vi "startReadSetDuration.vi"(8 "error in (no error)":errorcluster, 9 "duration":dbl, 10 "ElectrometerController in":refnum<class "ElectrometerController.lvclass">, 11 "State in":refnum<class "State.lvclass">) -> (0 "error out":errorcluster, 2 "ElectrometerController. out":refnum<class "ElectrometerController.lvclass">, 3 "State out":refnum<class "State.lvclass">)   [LabVIEW 2016, in "State.lvclass"]
uses:
  State.lvclass
  ElectrometerController/ElectrometerController.lvclass
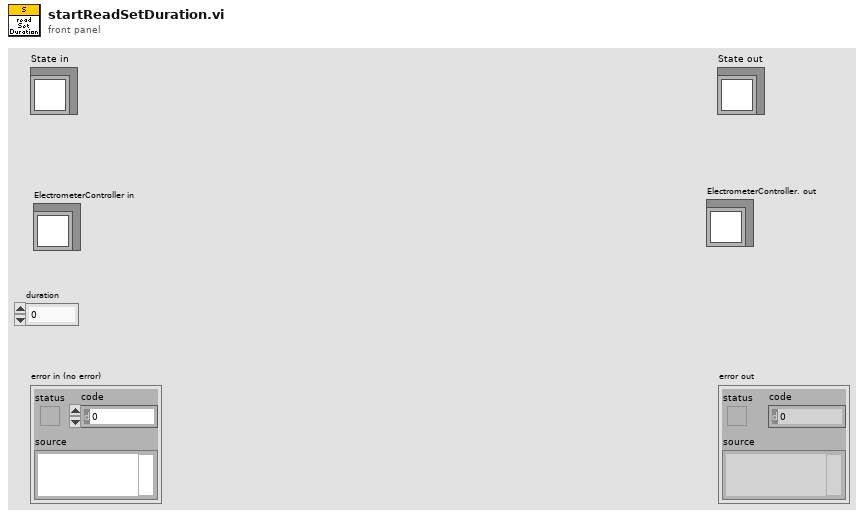
[diagram p1: front panel]
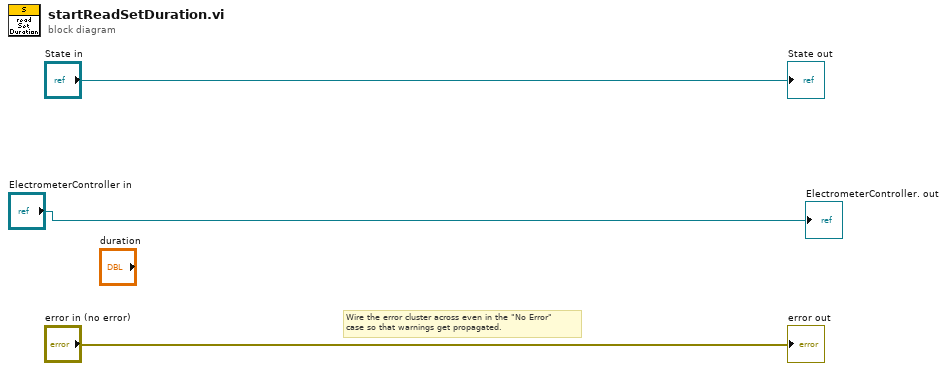
[diagram p0: block diagram]
diagram:
  # "Wire the error cluster across even in the \"No Error\"\ncase so that warnings get propagated."
  "error out" <- "error in (no error)"
  "State out" <- "State in"
  "ElectrometerController. out" <- "ElectrometerController in"
